vi "MRC Configure.vi"(8 "error in (no error)":errorcluster, 10 "Message Data":variant, 11 "Data Cluster":T2={"MFC Definition"={"MFC Port"="", "MFC Enable"=TRUE, "Baud Rate"=0, "Interface type"=enum."RS-485", "Address"=0}, "Set Point Options"={"Setpoint Value"=0.0, "Mass Flow EU 2"="", "Setpoint Source"="", "Valve Mode"=""}, "Writer Queue"=refnum, "Enable"=FALSE, "Update Rate"=0, "MRC Chamber Enable"=FALSE, "Selected Gas"="", "Address String"=""} {"Set Point Options"."Setpoint Value" min=0.0 max=0.62495 format="%.5f"}) -> (0 "error out":errorcluster, 1 "Message":T1, 2 "Send Resp":bool, 3 "Data Cluster out":T2={"MFC Definition"={"MFC Port"="", "MFC Enable"=TRUE, "Baud Rate"=0, "Interface type"=enum."RS-485", "Address"=0}, "Set Point Options"={"Setpoint Value"=0.0, "Mass Flow EU 2"="", "Setpoint Source"="", "Valve Mode"=""}, "Writer Queue"=refnum, "Enable"=FALSE, "Update Rate"=0, "MRC Chamber Enable"=FALSE, "Selected Gas"="", "Address String"=""} {"Set Point Options"."Setpoint Value" min=0.0 max=0.62495 format="%.5f"})   [LabVIEW 2020, in "MRC Module.lvlib"]
uses:
  MRC Module.lvlib
  MRC Configuration.ctl
  support/Message Queue/Message Cluster.ctl
  NCD Update Settings Setpoints.vi
  NCD Update Settings Valve.vi
  support/Message Queue/Message Queue.lvlib
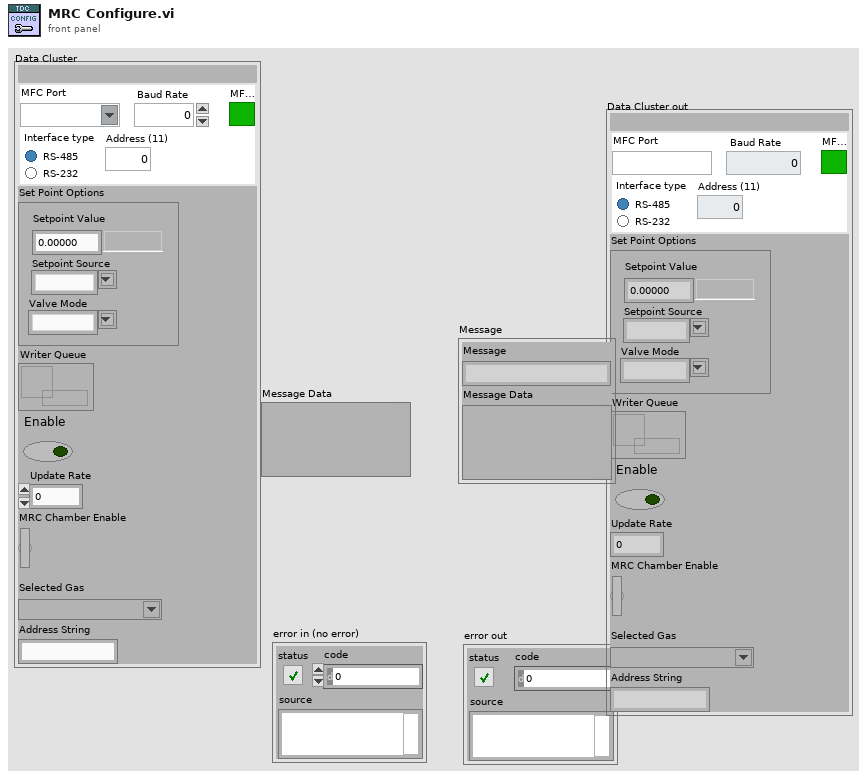
[diagram p1: front panel]
types:
  T1 = typedef "Message Queue.lvlib/Message Cluster.ctl" = cluster{"Message":string, "Message Data":variant}
  T2 = typedef "MRC Module.lvlib/MRC Configuration.ctl" = cluster{"MFC Definition":cluster{"MFC Port":refnum<visa-resource-name>, "MFC Enable":bool, "Baud Rate":i32, "Interface type":enum32{"RS-485", "RS-232"}, "Address":i32}, "Set Point Options":cluster{"Setpoint Value":dbl, "Mass Flow EU 2":string, "Setpoint Source":string, "Valve Mode":string}, "Writer Queue":refnum<queue>, "Enable":bool, "Update Rate":u32, "MRC Chamber Enable":bool, "Selected Gas":string, "Address String":string}
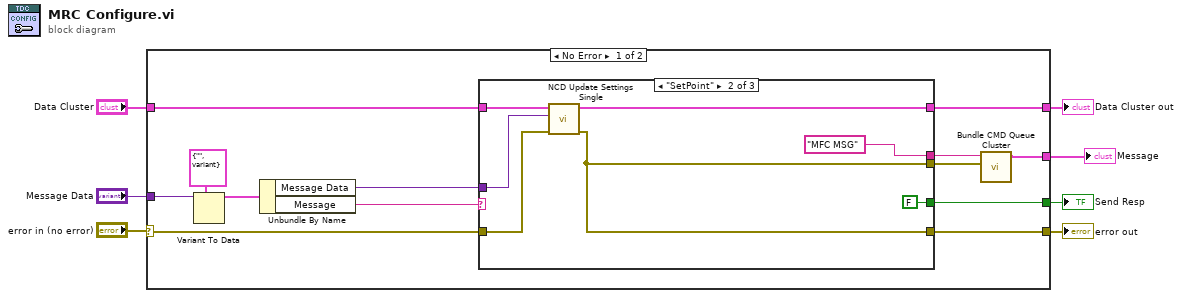
[diagram p0: block diagram]
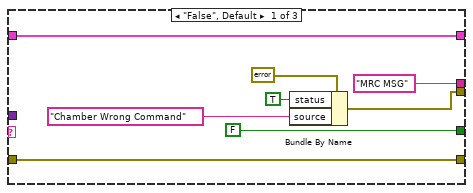
[diagram p2: hidden frame]
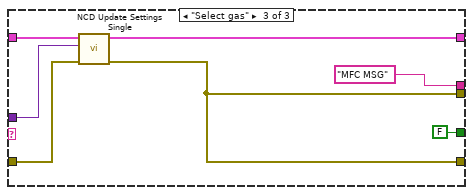
[diagram p3: hidden frame]
diagram:
  n1 = case shown="No Error" "error in (no error)" {
    selector: "error in (no error)" -> [w13 w43]
    tunnel: [w20 w43] -> w7
    tunnel: "Data Cluster" -> [w19 w44]
    tunnel: [w18 w44] -> w5
    tunnel: "Message Data" -> [w14 _]
    tunnel: [w12 _] -> w2
    tunnel: [w10 _] -> w1
    frame No Error {
      n2 = Variant To Data(type=T1 {"Message"="", "Message Data"=variant} ("element"), Variant=w14) -> (data=w16:T1)  [unwired: 1 in, 1 out]
      n3 = Unbundle By Name(w16) -> ("Message Data"=w11:variant, "Message"=w17:string)
      n4 = case shown="\"SetPoint\"" w17 {
        tunnel: w11 -> [_ w35 w42]
        tunnel: [w28 w32 w39] -> w18
        tunnel: w19 -> [w28 w33 w40]
        tunnel: w13 -> [w27 w34 w41]
        tunnel: [w27 w29 w36] -> w20
        tunnel: [FALSE ("Send Resp") FALSE ("Send Resp") FALSE ("Send Resp")] -> w12
        tunnel: [w21 w29 w36] -> w9
        tunnel: ["MRC MSG" ("Type CMD") "MFC MSG" ("Type CMD") "MFC MSG" ("Type CMD")] -> w8
        frame "False", Default {
          n5 = Bundle By Name(cluster=errorcluster {"status"=FALSE, "code"=0, "source"=""} ("error out"), "status"=TRUE, "source"="Chamber Wrong Command") -> (w21:errorcluster)
        }
        frame "SetPoint" {
          n6 = call-poly "NCD Update Settings Single.vi"("error in (no error)"=w34, "Message Data"=w35, "Data Cluster"=w33) -> ("error out"=w29:errorcluster, "Data Cluster out"=w32:T2)  [unwired: 5 in, 2 out]
        }
        frame "Select gas" {
          n7 = call-poly "NCD Update Settings Single.vi"("error in (no error)"=w41, "Message Data"=w42, "Data Cluster"=w40) -> ("error out"=w36:errorcluster, "Data Cluster out"=w39:T2)  [unwired: 6 in, 1 out]
        }
      }
      n8 = call "Bundle CMD Queue Cluster.vi"("Message Data"=w9, "Message"=w8) -> ("Message Cluster"=w10:T1)  [unwired: 9 in]
    }
    frame Error {
    }
  }
  "error out" <- w7
  "Data Cluster out" <- w5
  "Send Resp" <- w2
  "Message" <- w1
